vi "ShowMessage.vi"(6 "DefaultButton":u32(ring) items=["Button1"=0, "Button2"=256, "Button3"=512, "Button4"=768], 8 "IconOption":u32(ring)=10 items=["Stop/Error/Hand"=16, "Question"=32, "Warning/Exclamation"=48, "Information"=64], 9 "ButtonOption":u32(ring) items=["OK", "OK/Cancel", "Abort/Retry/Ignore", "Yes/No/Cancel", "Yes/No", "Retry/Cancel", "Cancel/TryAgain/Continue"], 10 "Captial":string, 11 "Message":string) -> (3 "ReturnValue":u32(ring) items=["RunError"=0, "OK"=1, "Cancel"=2, "Abort"=3, "Retry"=4, "Igonre"=5, "Yes"=6, "No"=7, "Try Again"=10, "Continue"=11])   [LabVIEW 2018]
doc: "调用系统MessageBox对话框。"
uses:
  user32.dll
panel:
  out "错误输出":errorcluster
  out "result":i32
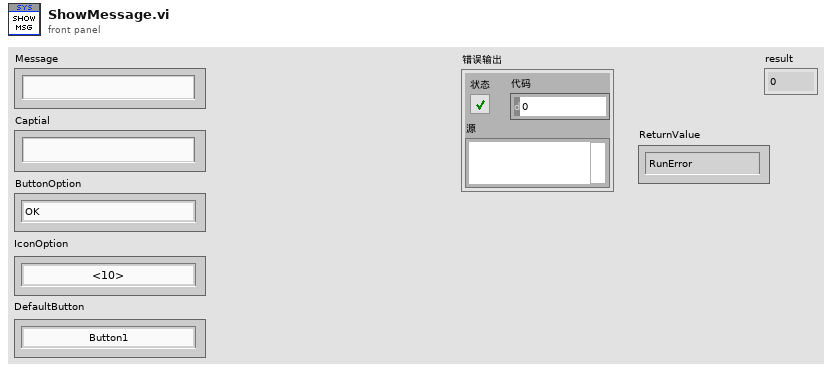
[diagram p1: front panel]
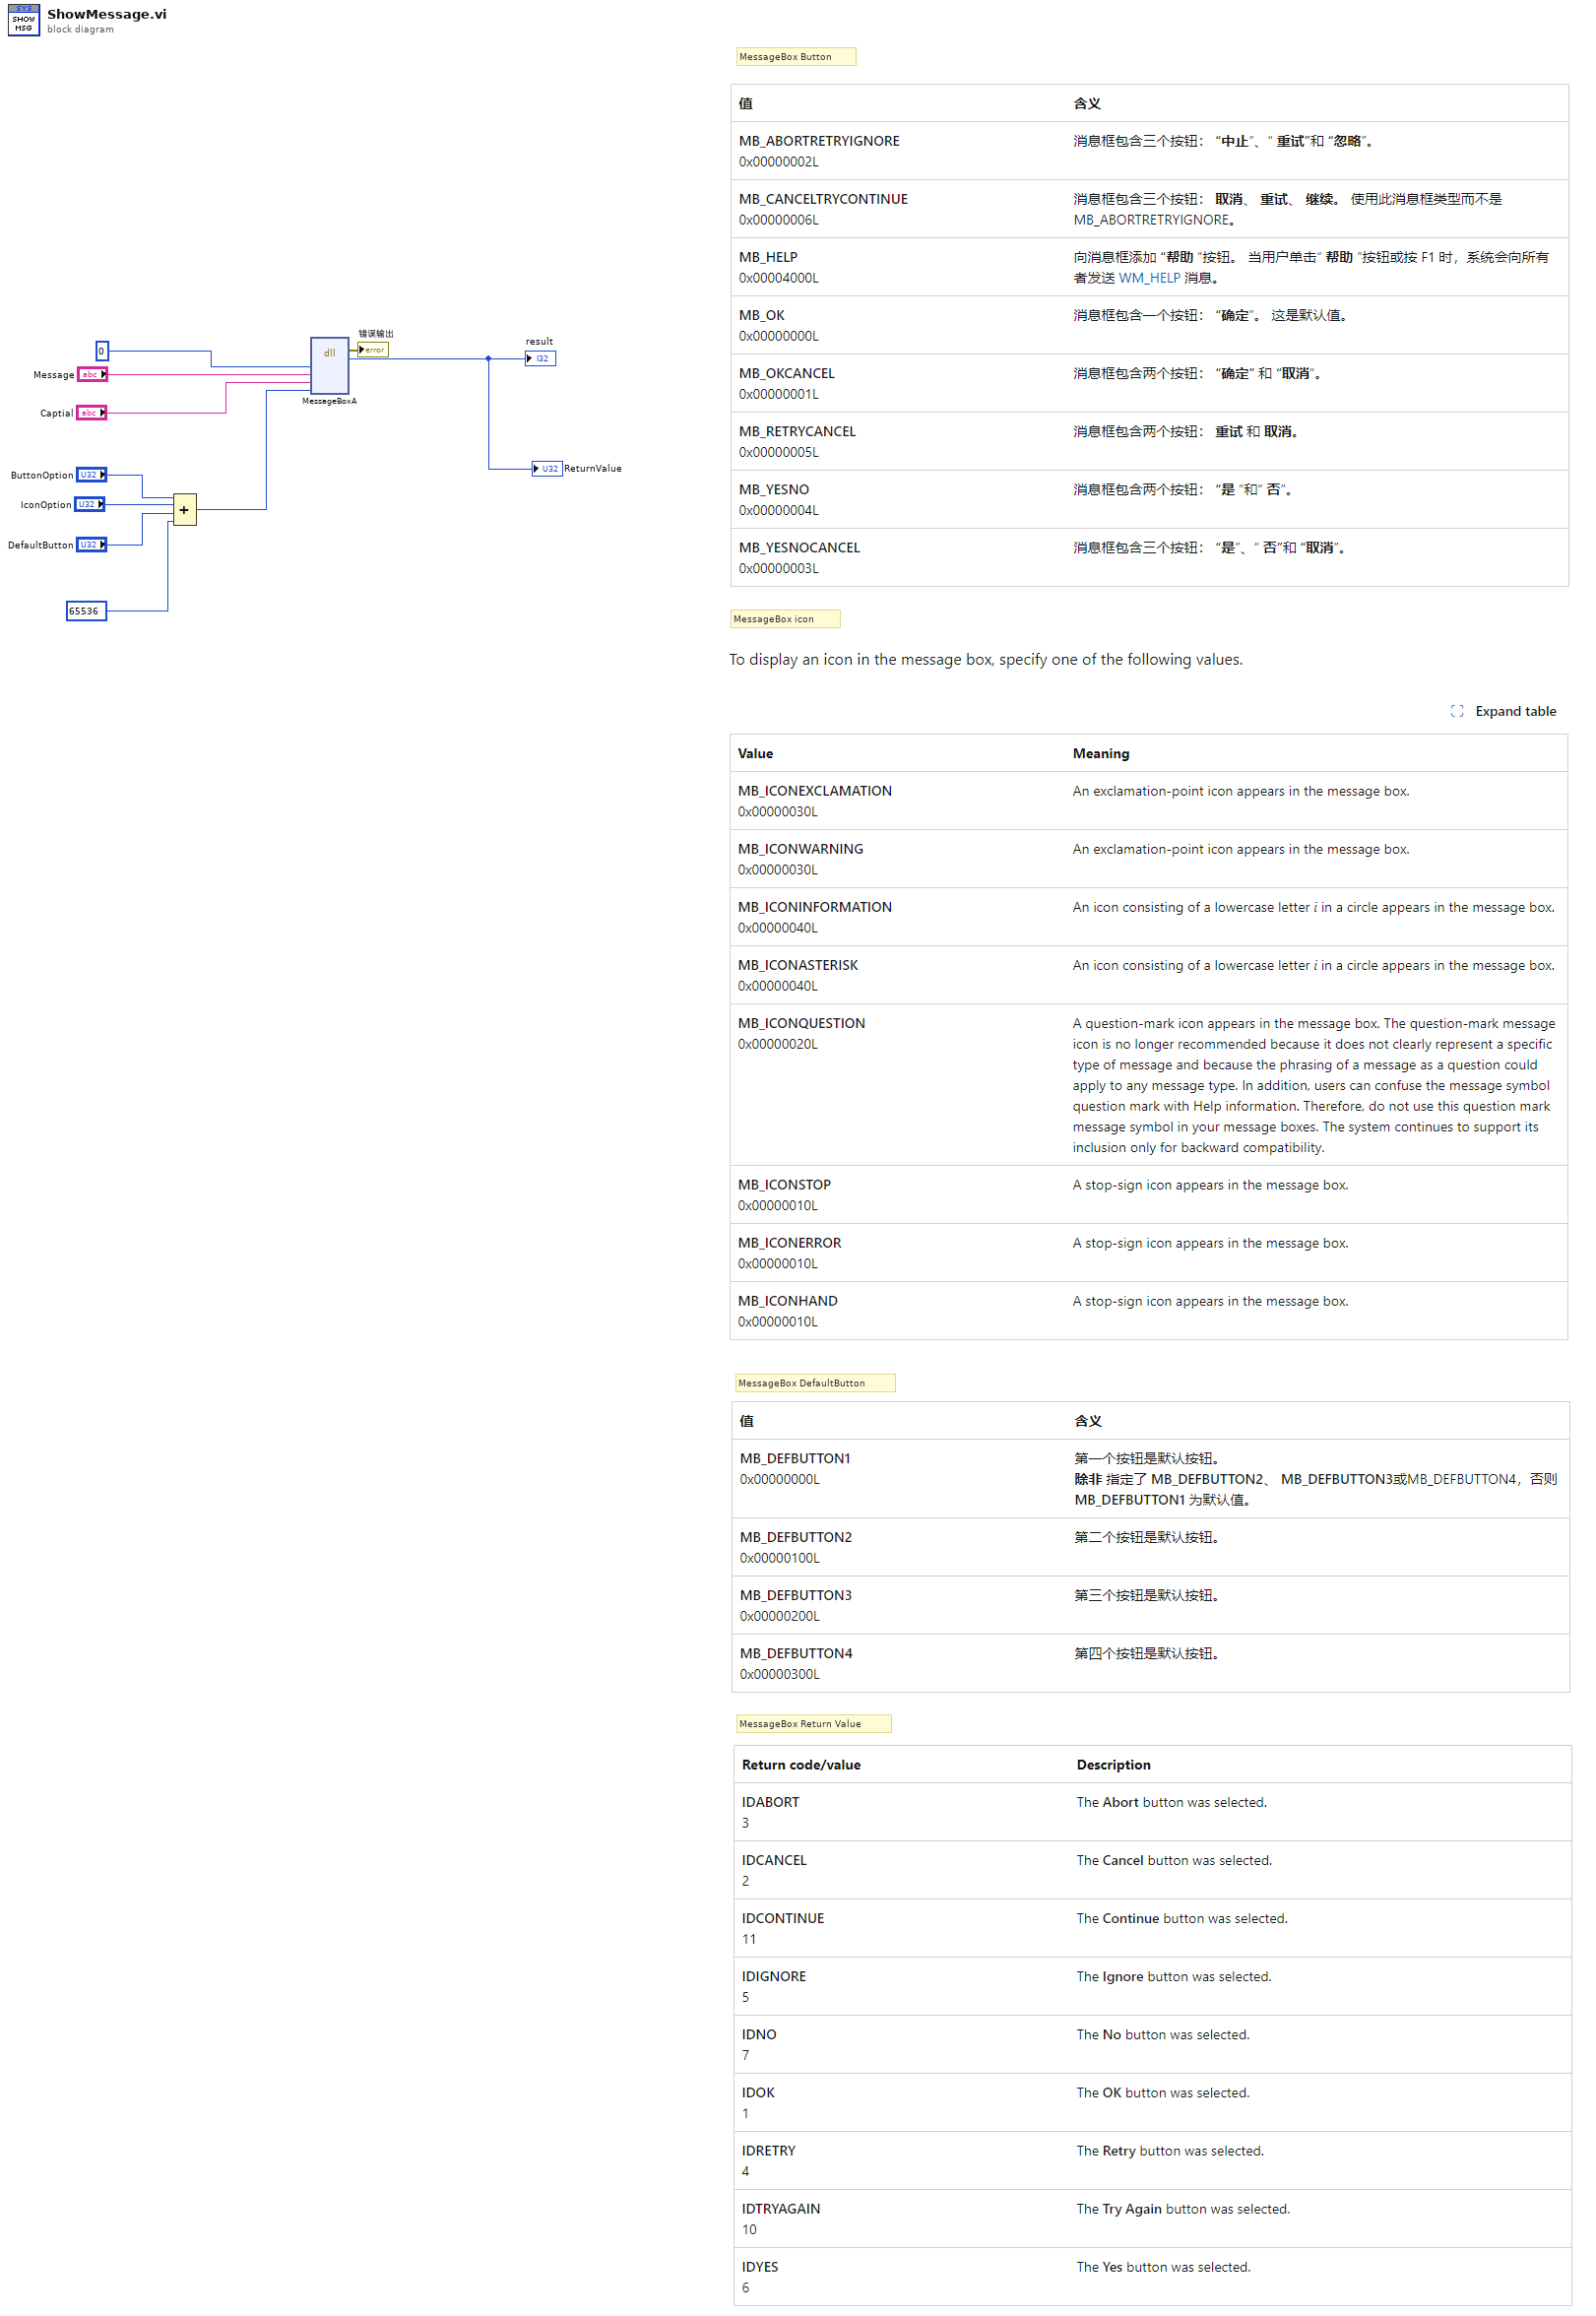
[diagram p0: block diagram]
diagram:
  # "MessageBox Return Value"
  # "MessageBox DefaultButton"
  # "MessageBox Button"
  # "MessageBox icon"
  n1 = Compound Arithmetic op=ADD("ButtonOption", "IconOption", "DefaultButton", u32 65536) -> (w4:u32)
  n2 = dll-call lib="user32.dll" fn="MessageBoxA"("Owner"=u64 0, "Message"="Message", "Captial"="Captial", "Mode"=w4) -> (error out=→"错误输出":errorcluster, "返回类型"=→"result" →"ReturnValue":i32)  [unwired: 7 in, 1 out]
